vi "ParseVectorFile.SVG.DotFactory.vi"(8 "error in (no error)":errorcluster, 11 "ParseVectorFile in":refnum<class "ParseVectorFile.lvclass">) -> (0 "error out":errorcluster, 3 "ParseVectorFile out":refnum<class "ParseVectorFile.lvclass">)   [LabVIEW 2019, in "ParseVectorFile.lvclass"]
uses:
  ParseVectorFile.lvclass
  ParseVectorFile.lvclass/ParseVectorFile.ctl
  ParseXML/ParseSVG.lvclass/ParseSVG.ctl
  Dot/Dot.lvclass
  Dot/CircleData.ctl
  ParseXML/ParseSVG.lvclass
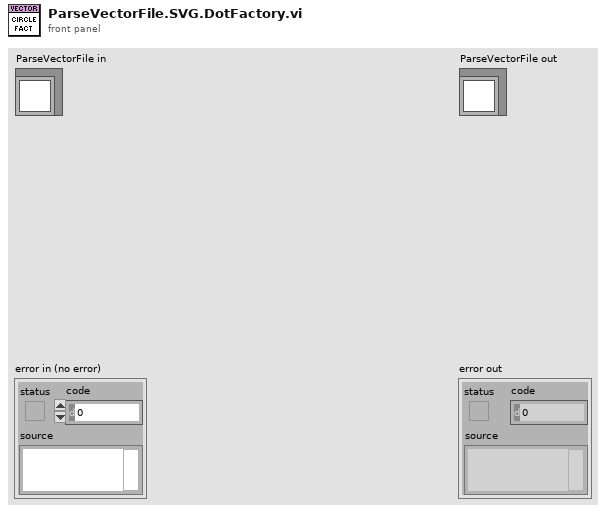
[diagram p1: front panel]
types:
  T1 = typedef "ParseSVG.lvclass/Dot.ctl" = cluster{"cx":string, "cy":string, "r":string, "style":string, "id":string}
  T2 = typedef "Dot.lvclass/CircleData.ctl" = cluster{"cx":string, "cy":string, "r":string}
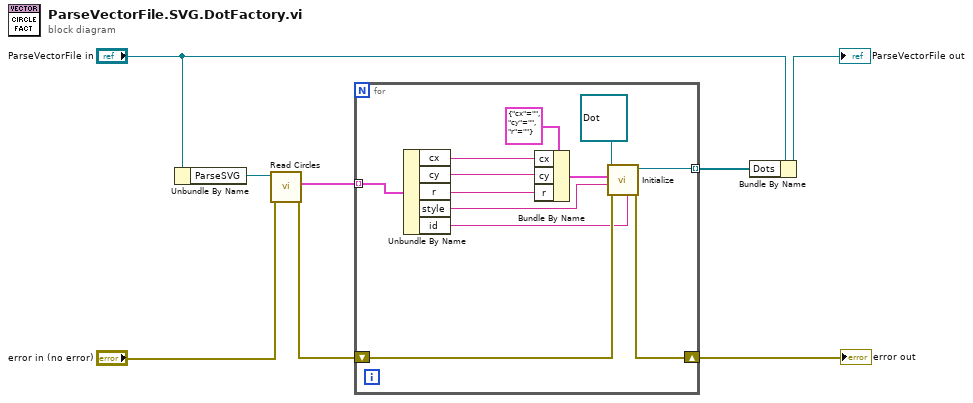
[diagram p0: block diagram]
diagram:
  n1 = Unbundle By Name("ParseVectorFile in") -> ("ParseSVG"=w8:refnum<class "ParseSVG.lvclass">)
  n2 = call "Read Circles.vi"("error in (no error)"="error in (no error)", "ParseSVG in"=w8) -> ("error out"=w5:errorcluster, "Circles"=w6:T1[])  [unwired: 7 in, 1 out]
  n3 = for {
    tunnel: w6 -> [w20] mode=indexing
    shift-right: [w12] -> w4
    shift-left: w5 -> [w13]
    tunnel: [w11] -> w3 mode=indexing
    n4 = Unbundle By Name(w20) -> ("cx"=w17:string, "cy"=w16:string, "r"=w15:string, "style"=w10:string, "id"=w9:string)
    n5 = Bundle By Name(cluster=T2 {"cx"="", "cy"="", "r"=""} ("Dot"), "cx"=w17, "cy"=w16, "r"=w15) -> (w14:T2)
    n6 = call "Initialize.vi"("id"=w9, "error in (no error)"=w13, "Style"=w10, "Dot"=w14, "Dot in"=refnum<class "Dot.lvclass"> refnum) -> ("error out"=w12:errorcluster, "Dot out"=w11:refnum<class "Dot.lvclass">)  [unwired: 5 in]
  }
  "error out" <- w4
  n7 = Bundle By Name(cluster="ParseVectorFile in", "Dots"=w3) -> (→"ParseVectorFile out":refnum<class "ParseVectorFile.lvclass">)
